vi "RemoveSubString.vi"(9 "Sub End":string, 10 "Sub Start":string, 11 "String In":string) -> (2 "Not Found?":bool, 3 "String Out":string)   [LabVIEW 2023]
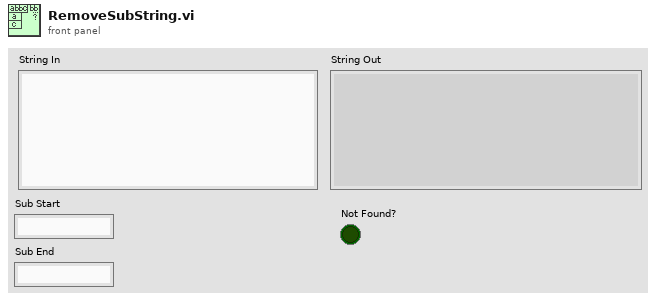
[diagram p1: front panel]
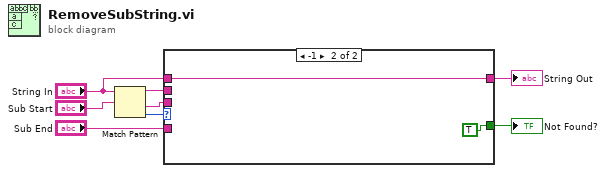
[diagram p0: block diagram]
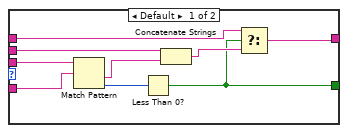
[diagram p2: hidden frame]
diagram:
  n1 = Match Pattern(string="String In", regular expression="Sub Start") -> (before substring=w3:string, after substring=w2:string, offset past match=w7:i32)  [unwired: 1 in, 1 out]
  n2 = case shown="-1" w7 {
    tunnel: [w9 w19] -> w6
    tunnel: "String In" -> [w12 w19]
    tunnel: [w10 TRUE] -> w4
    tunnel: w3 -> [w15 _]
    tunnel: w2 -> [w17 _]
    tunnel: "Sub End" -> [w16 _]
    frame Default {
      n3 = Match Pattern(string=w17, regular expression=w16) -> (after substring=w14:string, offset past match=w13:i32)  [unwired: 1 in, 2 out]
      n4 = Less Than 0?(x=w13) -> (x < 0?=w10:bool)
      n5 = Concatenate Strings(w15, w14) -> (w11:string)
      n6 = Select(t=w12, s=w10, f=w11) -> (s? t:f=w9:string)
    }
    frame -1 {
    }
  }
  "String Out" <- w6
  "Not Found?" <- w4
